vi "voltage out.vi"() -> ()   [LabVIEW 2009, in "Varian Magnet.lvclass"]
uses:
  Varian Magnet.lvclass
  <vilib>/DAQmx/write.llb/DAQmx Write (Analog DBL 1Chan 1Samp).vi
  <vilib>/DAQmx/create/channels.llb/DAQmx Create Channel (AO-Voltage-Basic).vi
panel:
  in  "stop":bool
  out "Numeric":dbl
  in  "data":dbl format="%0.2f"
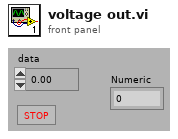
[diagram p1: front panel]
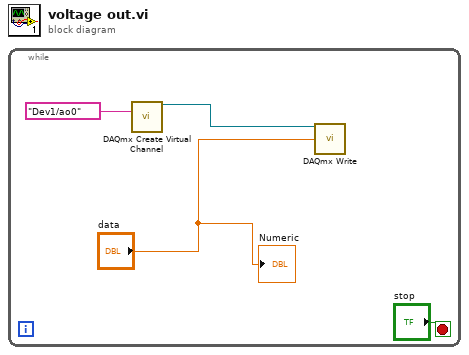
[diagram p0: block diagram]
diagram:
  n1 = while {
    stop <- "stop" stop-if-true
    n2 = call-poly <vilib>:"DAQmx Create Virtual Channel.vi"("physical channels"=tag "Dev1/ao0") -> ("task out"=w2:refnum<k21>)  [unwired: 13 in, 1 out]
    n3 = call-poly <vilib>:"DAQmx Write.vi"("task/channels in"=w2, "data"="data") -> ()  [unwired: 11 in, 3 out]
    "Numeric" <- "data"
  }
